vi "End Metric.vi"(5 "Start HRS":dbl format="%_19f", 7 "Metric":string, 8 "error in (no error)":errorcluster, 11 "Module in":refnum<class "Module.lvclass">) -> (0 "error out":errorcluster, 3 "Module out":refnum<class "Module.lvclass">, 9 "End HRS":dbl)   [LabVIEW 2020, in "Volatus.lvlib" / "Module.lvclass"]
uses:
  Module.lvclass
  Module.lvclass/Module.ctl
  MessageQ/MessageQ.lvclass/MessageQ.ctl
  Forward Metric.vi
  Parent Q.vi
  MessageQ/Is Null.vi
  MessageQ/Send.vi
  <vilib>/ptbypt/NI_PtbyPt.lvlib
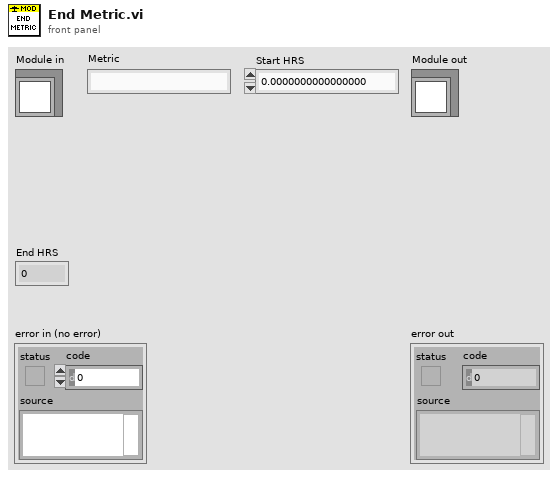
[diagram p1: front panel]
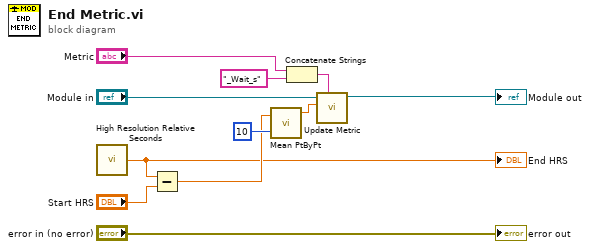
[diagram p0: block diagram]
diagram:
  n1 = call <vilib>:"High Resolution Relative Seconds.vi"() -> ("relative seconds"=w1:dbl)
  "End HRS" <- w1
  n2 = Subtract(x=w1, y="Start HRS") -> (x-y=w2:dbl)
  n3 = call <vilib>:"Mean PtByPt.vi"("x"=w2, "sample length"=10) -> ("mean"=w6:dbl)  [unwired: 2 in, 1 out]
  n4 = Concatenate Strings("Metric", "_Wait_s" ("string")) -> (w7:string)
  n5 = call "Update Metric.vi"("Metric"=w7, "Value"=w6, "Module in"="Module in") -> ("Module out"=→"Module out":refnum<class "Module.lvclass">)  [unwired: 7 in, 1 out]
  "error out" <- "error in (no error)"
